vi "login.vi"() -> ()   [LabVIEW 2020, in "userLibrary.lvlib"]
uses:
  userLibrary.lvlib
  <vilib>/measure/mamon.llb/Trigger Detection for 1 Channel.vi
  maintenanceLibrary.lvlib
  <vilib>/measure/NI_MAPro.lvlib
  databaseLibrary.lvlib
panel:
  out "status 2":bool
  out "status 1":bool
  in  "Remember Me":bool
  in  "Cancel":bool
  in  "OK":bool
  in  "Password":string
  in  "Username":string
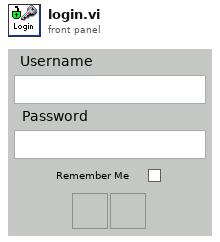
[diagram p1: front panel]
types:
  T1 = cluster{"string":string, "date/time string":string, "date/time string":string, string}
  T2 = cluster{i16, "date/time string":string, "date/time string":string, "Value":string, "Value":string}
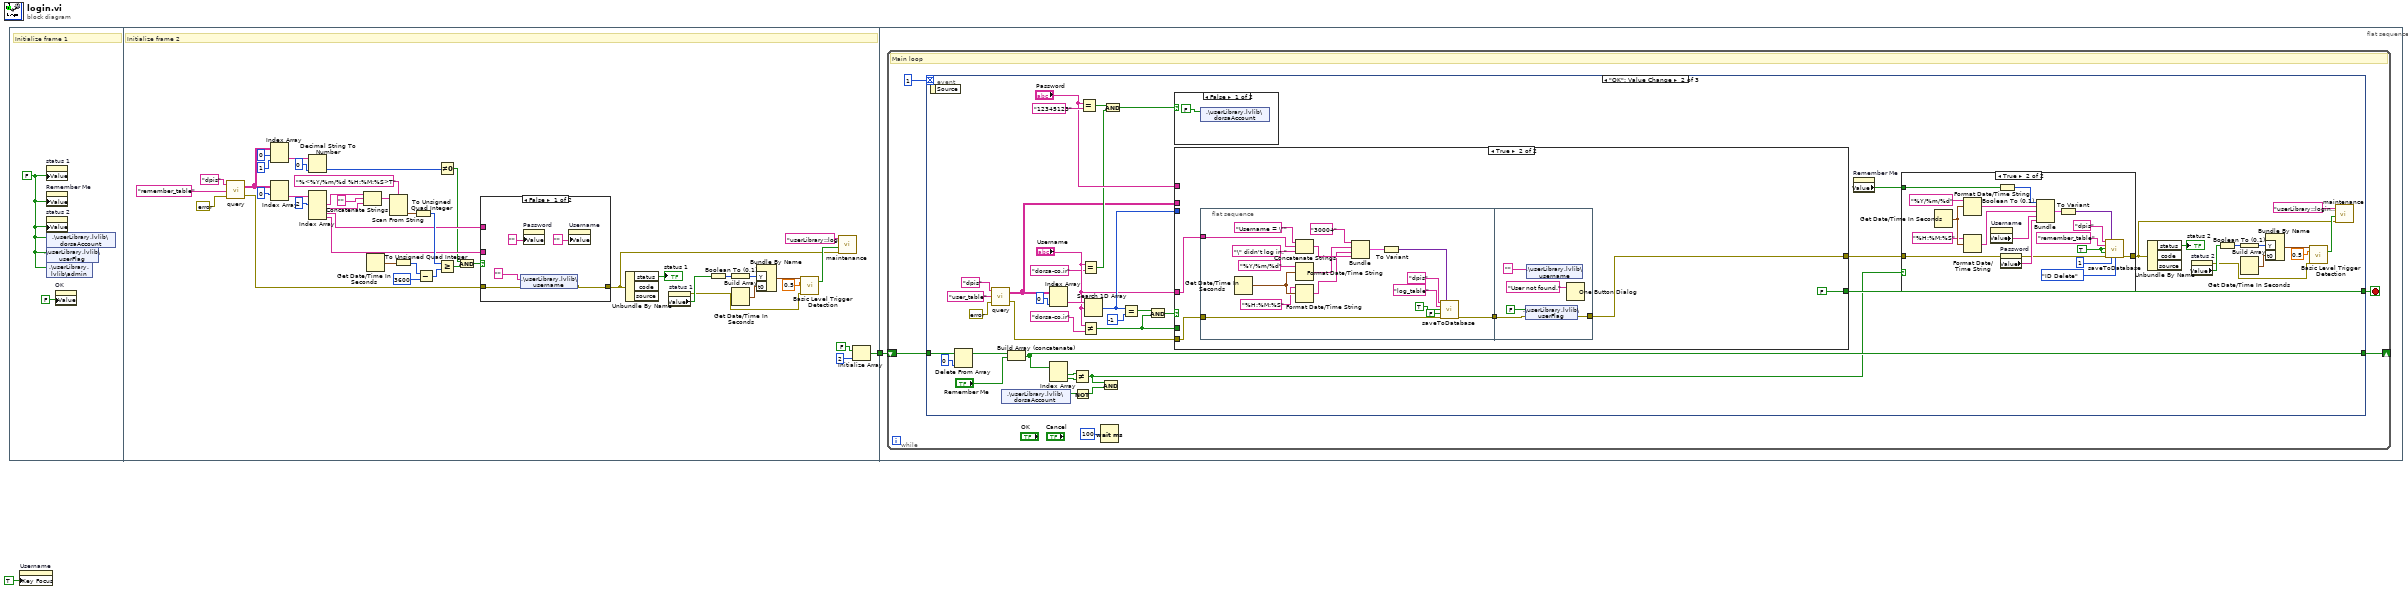
[diagram p0: block diagram]
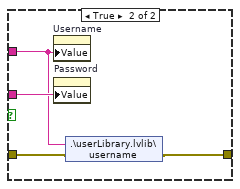
[diagram p2: hidden frame]
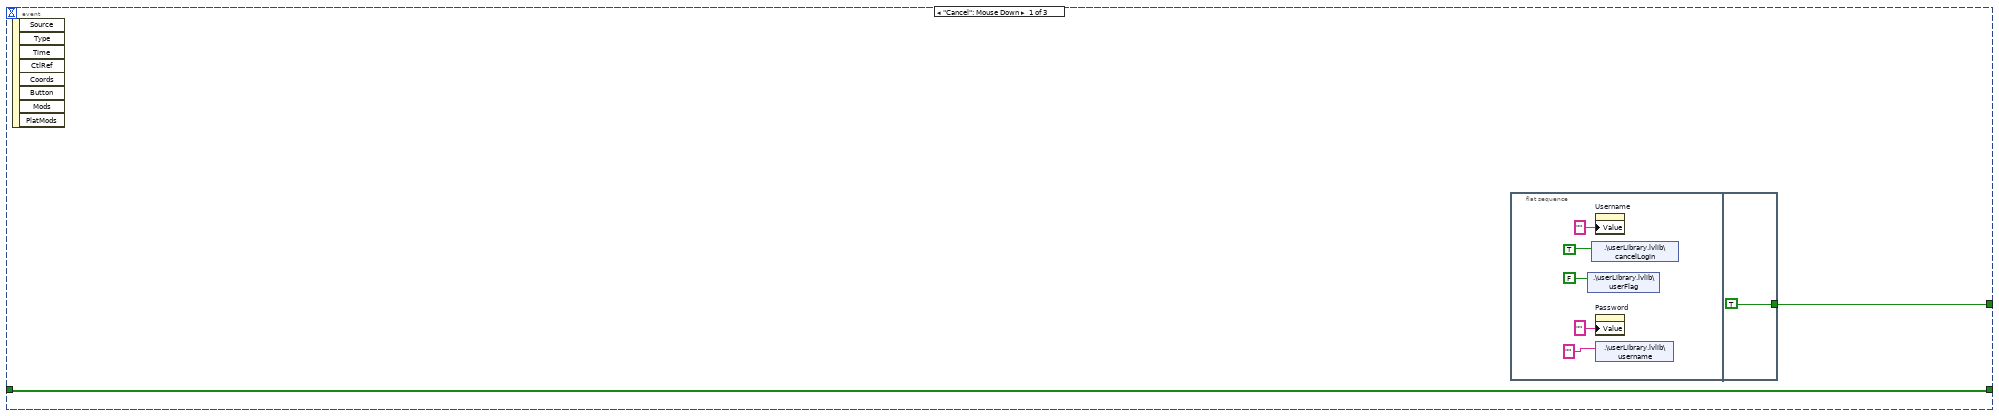
[diagram p3: hidden frame]
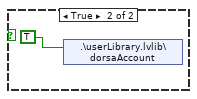
[diagram p5: hidden frame]
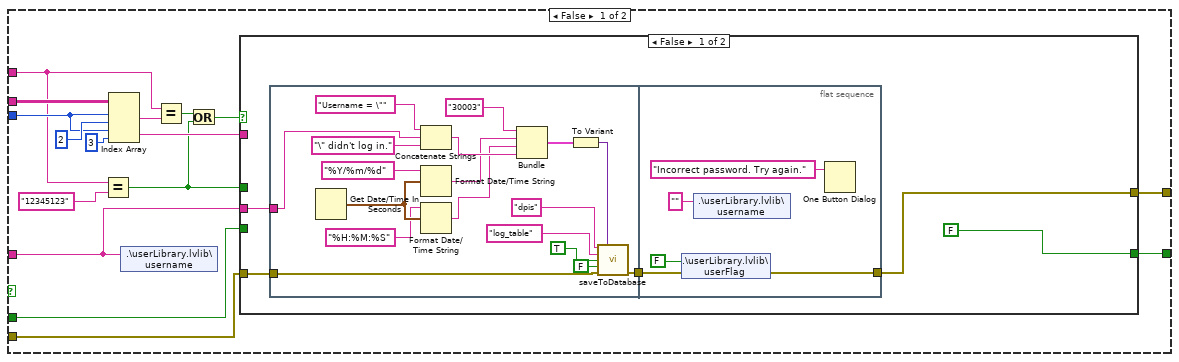
[diagram p6: hidden frame]
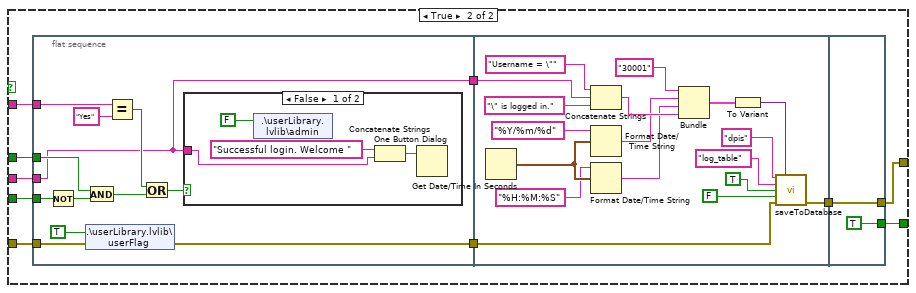
[diagram p7: hidden frame]
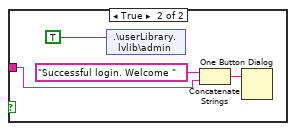
[diagram p8: hidden frame]
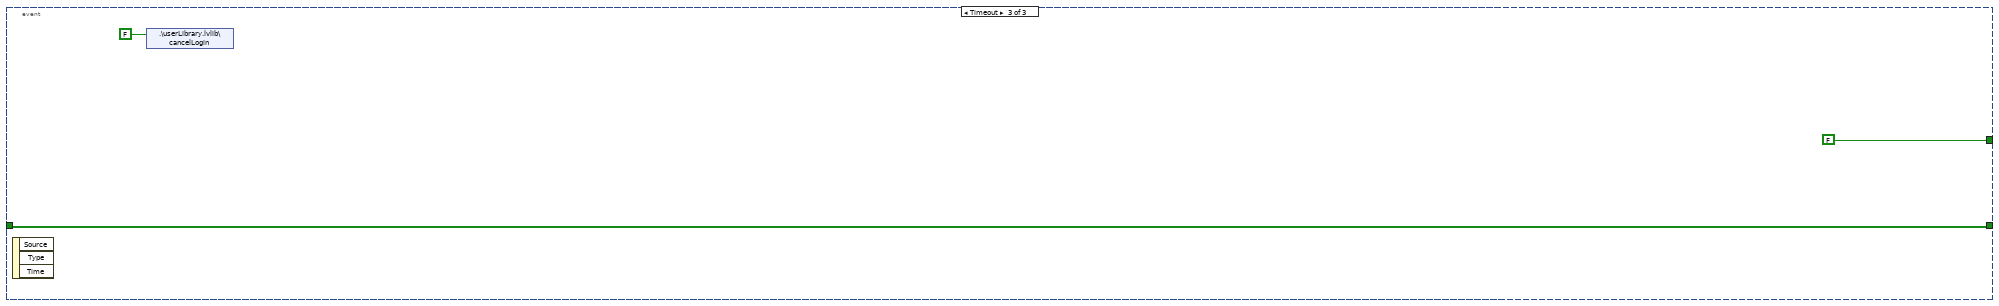
[diagram p9: hidden frame]
diagram:
  n1 = flat-sequence {
    tunnel: [w47] -> w1
    tunnel: w1 -> [w57]
    frame #0 {
      w4 = FALSE ("status 1")
      # "Initialize frame 1"
      n2 = property on="status 1" class="Bool (strict)"("Value"=w4) -> ()  [unwired: 2 in, 2 out]
      n3 = property on="Remember Me" class="Bool (strict)"("Value"=w4) -> ()  [unwired: 2 in, 2 out]
      n4 = property on="status 2" class="Bool (strict)"("Value"=w4) -> ()  [unwired: 2 in, 2 out]
      n5 = shared-variable ".\\userLibrary.lvlib\\dorsaAccount"(w4) -> ()  [unwired: 1 in, 1 out]
      n6 = shared-variable ".\\userLibrary.lvlib\\userFlag"(w4) -> ()  [unwired: 1 in, 1 out]
      n7 = shared-variable ".\\userLibrary.lvlib\\admin"(w4) -> ()  [unwired: 1 in, 1 out]
      n8 = property on="OK" class="Bool"("Value"=FALSE ("OK")) -> ()  [unwired: 2 in, 2 out]
    }
    frame #1 {
      # "Initialize frame 2"
      n9 = call "query.vi"("errorIn"=errorcluster {"status"=FALSE, "code"=0, "source"=""} ("Error in"), "Table Name"="remember_table", "Connection Name"="dpis") -> ("errorOut"=w6:errorcluster, "data"=w10:string[][])  [unwired: 1 in]
      n10 = Index Array(array=w10, index (row)=0, index (col)=1 ("disabled index (col)")) -> (element=w43:string)
      n11 = Index Array(array=w10, index (row)=0) -> (element=w39:string[])  [unwired: 1 in]
      n12 = Decimal String To Number(string=w43, default (0L)=u8 0 ("default (0 I32)")) -> (number=w41:u8)  [unwired: 1 in, 1 out]
      n13 = Index Array(array=w39, index #1=2 ("index")) -> (element #1=w36:string, element #2=w34:string, element #3=w27:string, element #4=w26:string)  [unwired: 3 in]
      n14 = Concatenate Strings(w36, "" ("string"), w34) -> (w33:string)
      n15 = Get Date/Time In Seconds() -> (seconds since 1Jan1904=w32:timestamp)
      n16 = Scan From String(format string="%<%Y/%m/%d %H:%M:%S>T", input string=w33) -> (output 1=w30:timestamp)  [unwired: 3 in, 3 out]
      n17 = To Unsigned Quad Integer(1:w32) -> (0:w31:u64)
      n18 = To Unsigned Quad Integer(1:w30) -> (0:w29:u64)
      n19 = Subtract(x=w31, y=u64 3600) -> (x-y=w28:u64)
      n20 = Not Equal To 0?(x=w41) -> (x != 0?=w23:bool)
      n21 = Greater Or Equal?(x=w29, y=w28) -> (x >= y?=w24:bool)
      n22 = And(x=w23, y=w24) -> (x .and. y?=w25:bool)
      n23 = case shown="False" w25 {
        tunnel: w27 -> [_ w55]
        tunnel: w26 -> [_ w56]
        tunnel: w6 -> [w49 w53]
        tunnel: [w50 w54] -> w11
        frame False {
          n24 = shared-variable ".\\userLibrary.lvlib\\username"("" ("Username"), error in=w49) -> (error out=w50:errorcluster)
          n25 = property on="Password" class="Str"("Value"="" ("Password")) -> ()  [unwired: 2 in, 2 out]
          n26 = property on="Username" class="Str"("Value"="" ("Username")) -> ()  [unwired: 2 in, 2 out]
        }
        frame True {
          n27 = property on="Username" class="Str"("Value"=w55) -> ()  [unwired: 2 in, 2 out]
          n28 = property on="Password" class="Str"("Value"=w56) -> ()  [unwired: 2 in, 2 out]
          n29 = shared-variable ".\\userLibrary.lvlib\\username"(w55, error in=w53) -> (error out=w54:errorcluster)
        }
      }
      n30 = Unbundle By Name(w11) -> ("status"=→"status 1":bool)  [unwired: 2 out]
      n31 = property on="status 1" class="Bool (strict)"() -> (error out=w14:errorcluster, "Value"=w15:bool)  [unwired: 2 in, 1 out]
      n32 = Boolean To (0,1)(Boolean=w15) -> (0, 1=w21:i16)
      n33 = Build Array(w21) -> (w19:i16[])
      n34 = Get Date/Time In Seconds() -> (seconds since 1Jan1904=w20:timestamp)
      n35 = Bundle By Name("Y"=w19, "t0"=w20) -> (w18:waveform(i16))  [unwired: 1 in]
      n36 = call-poly <vilib>:"Basic Level Trigger Detection.vi"("signal in"=w18, "level"=0.5, "error in (no error)"=w14) -> ("trigger detected?"=w16:bool)  [unwired: 10 in, 2 out]
      n37 = call "maintenance.vi"("errorIn"=w11, "status"=w16, "errorLocation"="userLibrary::login.vi::Initialize frame 2::status 1") -> ()  [unwired: 8 in, 1 out]
      n38 = Initialize Array(FALSE ("element"), 2 ("dimension size")) -> (w47:bool[])
    }
    frame #2 {
      n39 = while {
        shift-right: [w58] -> _
        shift-left: w57 -> [w59]
        stop <- w60 stop-if-true
        # "Main loop"
        n40 = event shown="[1] \"OK\": Value Change" {
          selector: _ -> [_ _ _]
          dyn-events: _ -> [_ _ _]
          timeout: 1 -> [_ _ _]
          tunnel: [w64 w99 FALSE] -> w60
          tunnel: w59 -> [w63 w98 w260]
          tunnel: [w63 w79 w260] -> w58
          event "Cancel": Mouse Down {
            n41 = event-data() -> ()  [unwired: 1 in, 8 out]
            n42 = flat-sequence {
              tunnel: [TRUE] -> w64
              frame #0 {
                n43 = shared-variable ".\\userLibrary.lvlib\\userFlag"(FALSE ("User Flag")) -> ()  [unwired: 1 in, 1 out]
                n44 = shared-variable ".\\userLibrary.lvlib\\cancelLogin"(TRUE ("Login Boolean")) -> ()  [unwired: 1 in, 1 out]
                n45 = property on="Username" class="Str"("Value"="" ("Username")) -> ()  [unwired: 2 in, 2 out]
                n46 = property on="Password" class="Str"("Value"="" ("Password")) -> ()  [unwired: 2 in, 2 out]
                n47 = shared-variable ".\\userLibrary.lvlib\\username"("" ("Username")) -> ()  [unwired: 1 in, 1 out]
              }
              frame #1 {
              }
            }
          }
          event "OK": Value Change {
            n48 = event-data() -> ()  [unwired: 1 in, 1 out]
            n49 = Delete From Array(array=w98, index=0) -> (array with subset deleted=w96:bool[])  [unwired: 1 in, 1 out]
            n50 = call "query.vi"("errorIn"=errorcluster {"status"=FALSE, "code"=0, "source"=""} ("Error in"), "Table Name"="user_table", "Connection Name"="dpis") -> ("errorOut"=w80:errorcluster, "data"=w94:string[][])  [unwired: 1 in]
            n51 = shared-variable ".\\userLibrary.lvlib\\dorsaAccount"() -> (w73:bool)  [unwired: 1 in, 1 out]
            n52 = Build Array (concatenate)(w96, "Remember Me") -> (w79:bool[])
            n53 = Index Array(array=w79) -> (element #1=w78:bool, element #2=w77:bool)  [unwired: 2 in]
            n54 = Index Array(array=w94, index (col)=0 ("disabled index (col)")) -> (element=w113:string[])  [unwired: 1 in]
            n55 = Not Equal?(x=w78, y=w77) -> (x != y?=w71:bool)
            n56 = Not(x=w73) -> (.not. x?=w72:bool)
            n57 = Equal?(x="Password", y="12345123") -> (x = y?=w101:bool)
            n58 = Equal?(x="Username", y="dorsa-co.ir") -> (x = y?=w102:bool)
            n59 = Not Equal?(x="Username", y="dorsa-co.ir") -> (x != y?=w107:bool)
            n60 = Search 1D Array(1D array=w113, element="Username") -> (index of element=w111:i32)  [unwired: 1 in]
            n61 = And(x=w71, y=w72) -> ()  [unwired: 1 out]
            n62 = And(x=w101, y=w102) -> (x .and. y?=w100:bool)
            n63 = Equal?(x=w111, y=-1) -> (x = y?=w109:bool)
            n64 = And(x=w109, y=w107) -> (x .and. y?=w108:bool)
            n65 = case shown="False" w100 {
              frame False {
                n66 = shared-variable ".\\userLibrary.lvlib\\dorsaAccount"(FALSE ("Is Dorsa?")) -> ()  [unwired: 1 in, 1 out]
              }
              frame True {
                n67 = shared-variable ".\\userLibrary.lvlib\\dorsaAccount"(TRUE ("Is Dorsa?")) -> ()  [unwired: 1 in, 1 out]
              }
            }
            n68 = case shown="True" w108 {
              tunnel: w94 -> [w152 _]
              tunnel: w111 -> [w148 _]
              tunnel: "Password" -> [w143 _]
              tunnel: "Username" -> [w137 w231]
              tunnel: w107 -> [w142 _]
              tunnel: [w140 FALSE] -> w99
              tunnel: w80 -> [w139 w234]
              tunnel: [w138 w232] -> w75
              frame False {
                n69 = Equal?(x=w143, y="12345123" ("x")) -> (x = y?=w141:bool)
                n70 = Index Array(array=w152, index (row) #1=w148, index (col) #1=2 ("disabled index (col)"), index (row) #2=w148, index (col) #2=3 ("index (col)")) -> (element #1=w150:string, element #2=w147:string)
                n71 = shared-variable ".\\userLibrary.lvlib\\username"(w137) -> ()  [unwired: 1 in, 1 out]
                n72 = Equal?(x=w143, y=w150) -> (x = y?=w146:bool)
                n73 = Or(x=w146, y=w141) -> (x .or. y?=w145:bool)
                n74 = case shown="False" w145 {
                  tunnel: w147 -> [_ w190]
                  tunnel: w142 -> [_ w189]
                  tunnel: w141 -> [_ w188]
                  tunnel: w137 -> [w156 w187]
                  tunnel: [FALSE w185] -> w140
                  tunnel: w139 -> [w155 w184]
                  tunnel: [w154 w182] -> w138
                  frame False {
                    n75 = flat-sequence {
                      tunnel: w156 -> [w161]
                      tunnel: w155 -> [w158]
                      tunnel: [w160] -> w153
                      tunnel: [w177] -> w154
                      tunnel: w153 -> [w176]
                      frame #0 {
                        n76 = Get Date/Time In Seconds() -> (seconds since 1Jan1904=w174:timestamp)
                        n77 = Concatenate Strings("Username = \"" ("string"), w161, "\" didn't log in." ("string")) -> (w175:string)
                        n78 = Format Date/Time String(time format string (%c)="%Y/%m/%d", seconds (now)=w174) -> (date/time string=w173:string)  [unwired: 1 in]
                        n79 = Format Date/Time String(time format string (%c)="%H:%M:%S", seconds (now)=w174) -> (date/time string=w172:string)  [unwired: 1 in]
                        n80 = Bundle("string"="30003", "date/time string"=w173, "date/time string"=w172, w175) -> (w171:T1)  [unwired: 1 in]
                        n81 = To Variant(anything=w171) -> (Variant=w163:variant)
                        n82 = call "saveToDatabase.vi"("Connection"="dpis" ("table"), "Data"=w163, "Table"="log_table" ("table"), "Auto Increment ID?"=TRUE, "Delete row?"=FALSE, "Error in"=w158) -> ("Error out"=w160:errorcluster)  [unwired: 9 in]
                      }
                      frame #1 {
                        n83 = shared-variable ".\\userLibrary.lvlib\\userFlag"(FALSE ("User Flag"), error in=w176) -> (error out=w177:errorcluster)
                        n84 = shared-variable ".\\userLibrary.lvlib\\username"("" ("Username")) -> ()  [unwired: 1 in, 1 out]
                        n85 = One Button Dialog(message="Incorrect password. Try again.") -> ()  [unwired: 1 in, 1 out]
                      }
                    }
                  }
                  frame True {
                    n86 = flat-sequence {
                      tunnel: w190 -> [w201]
                      tunnel: w189 -> [w196]
                      tunnel: w188 -> [w200]
                      tunnel: w187 -> [w194]
                      tunnel: [w194] -> w186
                      tunnel: w184 -> [w192]
                      tunnel: [w193] -> w183
                      tunnel: w186 -> [w219]
                      tunnel: w183 -> [w211]
                      tunnel: [w214] -> w181
                      tunnel: [TRUE] -> w185
                      tunnel: [w229] -> w182
                      tunnel: w181 -> [w229]
                      frame #0 {
                        n87 = Not(x=w196) -> (.not. x?=w195:bool)
                        n88 = shared-variable ".\\userLibrary.lvlib\\userFlag"(TRUE, error in=w192) -> (error out=w193:errorcluster)
                        n89 = And(x=w200, y=w195) -> (x .and. y?=w198:bool)
                        n90 = Equal?(x=w201, y="Yes") -> (x = y?=w199:bool)
                        n91 = Or(x=w199, y=w198) -> (x .or. y?=w197:bool)
                        n92 = case shown="False" w197 {
                          tunnel: w194 -> [w205 w209]
                          frame False {
                            n93 = shared-variable ".\\userLibrary.lvlib\\admin"(FALSE ("Is Admin?")) -> ()  [unwired: 1 in, 1 out]
                            n94 = Concatenate Strings("Successful login. Welcome " ("message"), w205) -> (w204:string)
                            n95 = One Button Dialog(message=w204) -> ()  [unwired: 1 in, 1 out]
                          }
                          frame True {
                            n96 = shared-variable ".\\userLibrary.lvlib\\admin"(TRUE ("Is Admin?")) -> ()  [unwired: 1 in, 1 out]
                            n97 = Concatenate Strings("Successful login. Welcome " ("message"), w209) -> (w208:string)
                            n98 = One Button Dialog(message=w208) -> ()  [unwired: 1 in, 1 out]
                          }
                        }
                      }
                      frame #1 {
                        n99 = Get Date/Time In Seconds() -> (seconds since 1Jan1904=w227:timestamp)
                        n100 = Concatenate Strings("Username = \"" ("string"), w219, "\" is logged in." ("string")) -> (w228:string)
                        n101 = Format Date/Time String(time format string (%c)="%Y/%m/%d", seconds (now)=w227) -> (date/time string=w226:string)  [unwired: 1 in]
                        n102 = Format Date/Time String(time format string (%c)="%H:%M:%S", seconds (now)=w227) -> (date/time string=w225:string)  [unwired: 1 in]
                        n103 = Bundle("string"="30001", "date/time string"=w226, "date/time string"=w225, w228) -> (w224:T1)  [unwired: 1 in]
                        n104 = To Variant(anything=w224) -> (Variant=w215:variant)
                        n105 = call "saveToDatabase.vi"("Connection"="dpis" ("table"), "Data"=w215, "Table"="log_table" ("table"), "Auto Increment ID?"=TRUE, "Delete row?"=FALSE, "Error in"=w211) -> ("Error out"=w214:errorcluster)  [unwired: 9 in]
                      }
                      frame #2 {
                      }
                    }
                  }
                }
              }
              frame True {
                n106 = flat-sequence {
                  tunnel: w234 -> [w236]
                  tunnel: [w239] -> w233
                  tunnel: w231 -> [w238]
                  tunnel: w233 -> [w255]
                  tunnel: [w254] -> w232
                  frame #0 {
                    n107 = Get Date/Time In Seconds() -> (seconds since 1Jan1904=w252:timestamp)
                    n108 = Concatenate Strings("Username = \"" ("string"), w238, "\" didn't log in." ("string")) -> (w253:string)
                    n109 = Format Date/Time String(time format string (%c)="%Y/%m/%d", seconds (now)=w252) -> (date/time string=w251:string)  [unwired: 1 in]
                    n110 = Format Date/Time String(time format string (%c)="%H:%M:%S", seconds (now)=w252) -> (date/time string=w250:string)  [unwired: 1 in]
                    n111 = Bundle("string"="30004", "date/time string"=w251, "date/time string"=w250, w253) -> (w249:T1)  [unwired: 1 in]
                    n112 = To Variant(anything=w249) -> (Variant=w241:variant)
                    n113 = call "saveToDatabase.vi"("Connection"="dpis" ("table"), "Data"=w241, "Table"="log_table" ("table"), "Auto Increment ID?"=TRUE, "Delete row?"=FALSE, "Error in"=w236) -> ("Error out"=w239:errorcluster)  [unwired: 9 in]
                  }
                  frame #1 {
                    n114 = shared-variable ".\\userLibrary.lvlib\\userFlag"(FALSE ("User Flag"), error in=w255) -> (error out=w254:errorcluster)
                    n115 = shared-variable ".\\userLibrary.lvlib\\username"("" ("Username")) -> ()  [unwired: 1 in, 1 out]
                    n116 = One Button Dialog(message="User not found.") -> ()  [unwired: 1 in, 1 out]
                  }
                }
              }
            }
            n117 = property on="Remember Me" class="Bool (strict)"() -> ("Value"=w74:bool)  [unwired: 2 in, 2 out]
            n118 = case shown="True" w71 {
              tunnel: w74 -> [_ w126]
              tunnel: [w115 w120] -> w76
              tunnel: w75 -> [w115 w117]
              frame False {
              }
              frame True {
                w116 = TRUE ("Auto Increment ID?")
                n119 = Get Date/Time In Seconds() -> (seconds since 1Jan1904=w134:timestamp)
                n120 = Format Date/Time String(time format string (%c)="%Y/%m/%d", seconds (now)=w134) -> (date/time string=w131:string)  [unwired: 1 in]
                n121 = Format Date/Time String(time format string (%c)="%H:%M:%S", seconds (now)=w134) -> (date/time string=w130:string)  [unwired: 1 in]
                n122 = property on="Username" class="Str"() -> ("Value"=w128:string)  [unwired: 2 in, 2 out]
                n123 = Boolean To (0,1)(Boolean=w126) -> (0, 1=w125:i16)
                n124 = property on="Password" class="Str"(error in=w117) -> (error out=w122:errorcluster, "Value"=w127:string)  [unwired: 1 in, 1 out]
                n125 = Bundle(w125, "date/time string"=w131, "date/time string"=w130, "Value"=w128, "Value"=w127) -> (w129:T2)  [unwired: 1 in]
                n126 = To Variant(anything=w129) -> (Variant=w118:variant)
                n127 = call "saveToDatabase.vi"("Connection"="dpis", "Data"=w118, "Table"="remember_table", "Auto Increment ID?"=w116, "Delete row?"=w116, "Error in"=w122, "Maximum Row"=1, "Delete Method"=enum16{"ID Delete", "Time Delete"}."ID Delete") -> ("Error out"=w120:errorcluster)  [unwired: 7 in]
              }
            }
            n128 = Unbundle By Name(w76) -> ("status"=→"status 2":bool)  [unwired: 2 out]
            n129 = property on="status 2" class="Bool (strict)"() -> (error out=w83:errorcluster, "Value"=w84:bool)  [unwired: 2 in, 1 out]
            n130 = Boolean To (0,1)(Boolean=w84) -> (0, 1=w90:i16)
            n131 = Build Array(w90) -> (w88:i16[])
            n132 = Get Date/Time In Seconds() -> (seconds since 1Jan1904=w89:timestamp)
            n133 = Bundle By Name("Y"=w88, "t0"=w89) -> (w87:waveform(i16))  [unwired: 1 in]
            n134 = call-poly <vilib>:"Basic Level Trigger Detection.vi"("signal in"=w87, "level"=0.5, "error in (no error)"=w83) -> ("trigger detected?"=w85:bool)  [unwired: 10 in, 2 out]
            n135 = call "maintenance.vi"("errorIn"=w76, "status"=w85, "errorLocation"="userLibrary::login.vi::OK case") -> ()  [unwired: 8 in, 1 out]
          }
          event Timeout {
            n136 = event-data() -> ()  [unwired: 1 in, 3 out]
            n137 = shared-variable ".\\userLibrary.lvlib\\cancelLogin"(FALSE ("Login Boolean")) -> ()  [unwired: 1 in, 1 out]
          }
        }
        n138 = Wait (ms)(milliseconds to wait=u32 100) -> ()  [unwired: 1 out]
      }
    }
  }
  n139 = property on="Username" class="Str"("Key Focus"=TRUE) -> ()  [unwired: 2 in, 2 out]
